vi "zher2 - Hermitian Matrix Rank-2 Update (CDB).vi"(6 "alpha":cdb=1.0+0.0i, 8 "matrix A type":T1=3 items=["Lower Triangular"=2, "Upper Triangular"=3], 9 "A":T2, 10 "y":cdb[](array[numeric]), 11 "x":cdb[](array[numeric])) -> (0 "error":i32, 3 "zher2":T2)   [LabVIEW 2020, in "NI_AALBLAS.lvlib"]
doc: "Calculates the rank-2 update of the upper or lower triangular component of a Hermitian matrix."
uses:
  NI_AALBLAS.lvlib
  ComplexMatrix.ctl
  LV_UpLo.ctl
  Order.ctl
  Fucntion.ctl
  NI_Matrix.lvlib
panel:
  # "zher2=alpha*x*conjg(y')+conjg(alpha)*y*conjg(x')+A"
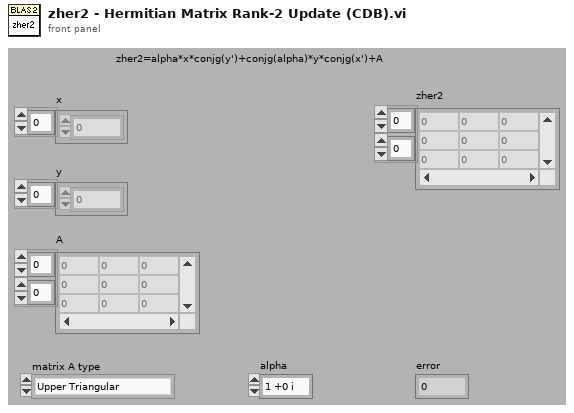
[diagram p1: front panel]
types:
  T1 = typedef "NI_AALBLAS.lvlib/LV_UpLo.ctl" = i32
  T2 = typedef "NI_Matrix.lvlib/ComplexMatrix.ctl" = cdb[][]
  T3 = typedef "NI_AALBLAS.lvlib/Fucntion.ctl" = u16
  T4 = typedef "NI_AALBLAS.lvlib/Order.ctl" = i32
  T5 = typedef "NI_AALBLAS.lvlib/UpLo.ctl" = i32
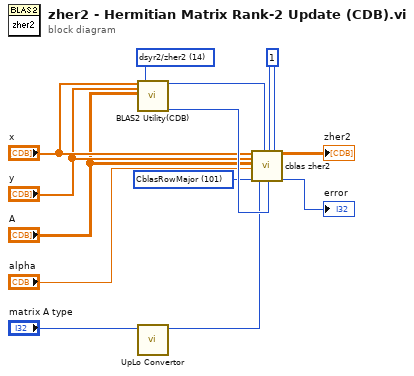
[diagram p0: block diagram]
diagram:
  w1 = 1
  w6 = T3 14 items=["ddot/zdotu/zdotc", "daxpy/zaxpy", "dnrm2/dznrm2", "dasum/dzasum", "dcopy/zcopy", "dswap/zswap", "drotm", "drot/zdrot", "idamax/izamax", "idamin/izamin", "dgemv/zgemv", "dsymv/zhemv", "dtrmv/ztrmv", "dsyr/zher", "dsyr2/zher2", "dger/zgeru/zgerc", "dtrsv/ztrsv", "dgemm/zgemm", "dsymm/zsymm/zhemm", "dtrmm/ztrmm", "dsyrk/zsyrk/zherk", "dsyr2k/zsyr2k/zher2k", "dtrsm/ztrsm"] ("function")
  w7 = T4 101 items=["CblasRowMajor"=101, "CblasColMajor"=102] ("order")
  n1 = call "BLAS2 Utility(CDB).vi"("x"="x", "y"="y", "A"="A", "function"=w6) -> ("lda"=w2:i32, "n"=w13:i32)  [unwired: 13 in, 1 out]
  n2 = call "UpLo Convertor.vi"("triangle matrix type"="matrix A type") -> ("uplo"=w10:T5)  [unwired: 10 out]
  n3 = call "cblas zher2.vi"("x"="x", "y"="y", "A"="A", "alpha"="alpha", "order"=w7, "uplo"=w10, "lda"=w2, "incx"=w1, "n"=w13, "incy"=w1) -> ("zher2"=→"zher2":T2, "error"=→"error":i32)  [unwired: 8 out]
